vi "updateCOMSettings.vi"(6 "timeout":i32=1500, 8 "error in (no error)":errorcluster, 9 "port":u16=50000, 10 "IP":string="127.0.0.1", 11 "AlCS in":refnum<class "AlCS.lvclass">) -> (0 "error out":errorcluster, 3 "AlCS out":refnum<class "AlCS.lvclass">)   [LabVIEW 2016, in "AlCS.lvclass"]
uses:
  AlCS.lvclass
  AlCS.lvclass/AlCS.ctl
  ts_labview_tcp/TCPClient/TCPClient.lvclass
  ts_labview_tcp/TCPSettings/TCPSettings.lvclass
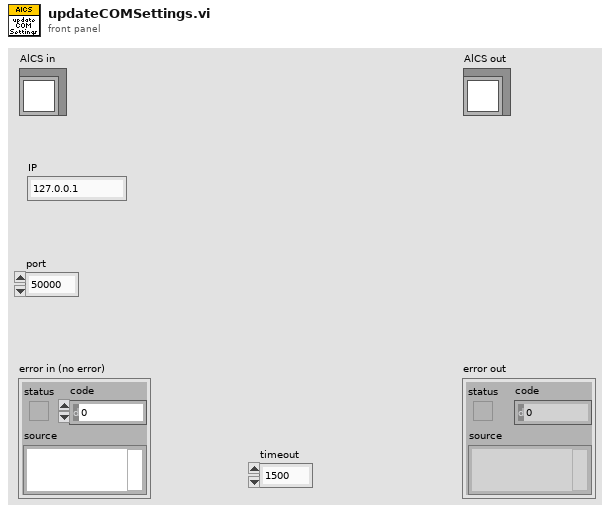
[diagram p1: front panel]
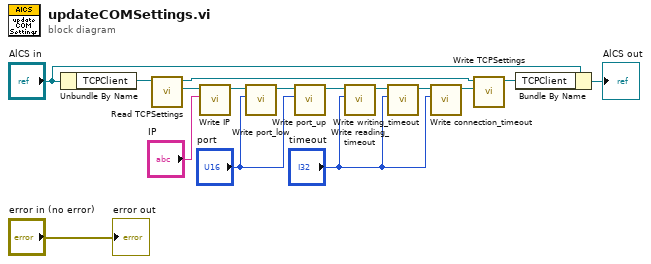
[diagram p0: block diagram]
diagram:
  n1 = Unbundle By Name("AlCS in") -> ("TCPClient"=w15:refnum<class "TCPClient.lvclass">)
  n2 = call-dynamic "Read TCPSettings.vi"("TCPCommunicator in"=w15) -> ("TCPSettings.lvclass"=w10:refnum<class "TCPSettings.lvclass">, "TCPCommunicator out"=w11:refnum<class "TCPClient.lvclass">)  [unwired: 8 in, 1 out]
  n3 = call-dynamic "Write IP.vi"("IP"="IP", "TCPSettings in"=w10) -> ("TCPSettings out"=w9:refnum<class "TCPSettings.lvclass">)  [unwired: 8 in, 1 out]
  n4 = call-dynamic "Write port_low.vi"("port_low"="port", "TCPSettings in"=w9) -> ("TCPSettings out"=w8:refnum<class "TCPSettings.lvclass">)  [unwired: 8 in, 1 out]
  n5 = call-dynamic "Write port_up.vi"("port_up"="port", "TCPSettings in"=w8) -> ("TCPSettings out"=w5:refnum<class "TCPSettings.lvclass">)  [unwired: 8 in, 1 out]
  n6 = call-dynamic "Write reading_timeout.vi"("reading_timeout"="timeout", "TCPSettings in"=w5) -> ("TCPSettings out"=w4:refnum<class "TCPSettings.lvclass">)  [unwired: 8 in, 1 out]
  n7 = call-dynamic "Write writing_timeout.vi"("writing_timeout"="timeout", "TCPSettings in"=w4) -> ("TCPSettings out"=w3:refnum<class "TCPSettings.lvclass">)  [unwired: 8 in, 1 out]
  n8 = call-dynamic "Write connection_timeout .vi"("connection_timeout"="timeout", "TCPSettings in"=w3) -> ("TCPSettings out"=w2:refnum<class "TCPSettings.lvclass">)  [unwired: 8 in, 1 out]
  n9 = call-dynamic "Write TCPSettings.vi"("TCPSettings.lvclass"=w2, "TCPCommunicator in"=w11) -> ("TCPCommunicator out"=w14:refnum<class "TCPClient.lvclass">)  [unwired: 8 in, 1 out]
  n10 = Bundle By Name(cluster="AlCS in", "TCPClient"=w14) -> (→"AlCS out":refnum<class "AlCS.lvclass">)
  "error out" <- "error in (no error)"
